vi "Interface.Set Response FIFO.vi"(10 "Response FIFO":T1, 11 "Interface in":refnum<class "Interface.lvclass">) -> (3 "Interface out":refnum<class "Interface.lvclass">)   [LabVIEW 2017, in "DSF Core.lvlib" / "Interface.lvclass"]
uses:
  Interface.lvclass
  Interface.RT FIFO.Ref.16B.ctl
  Interface.RT FIFO.Data.16B.ctl
  Interface.RT FIFO.Payload.16B.ctl
  Interface.lvclass/Interface.ctl
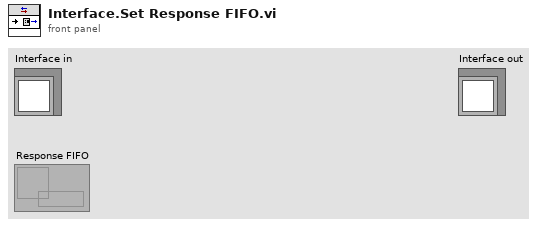
[diagram p1: front panel]
types:
  T1 = typedef "DSF Core.lvlib/Interface.lvclass/Interface.RT FIFO.Ref.16B.ctl" = refnum<k33>
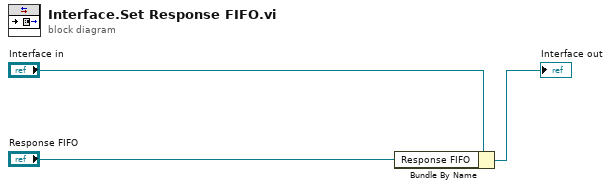
[diagram p0: block diagram]
diagram:
  n1 = Bundle By Name(cluster="Interface in", "Response FIFO"="Response FIFO") -> (→"Interface out":refnum<class "Interface.lvclass">)
